vi "ex02.vi"() -> ()   [LabVIEW 2011]
panel:
  in  "stop":bool
  out "Numeric 4":dbl
  out "Numeric 3":i64
  in  "Numeric 2":dbl
  in  "Numeric":i64
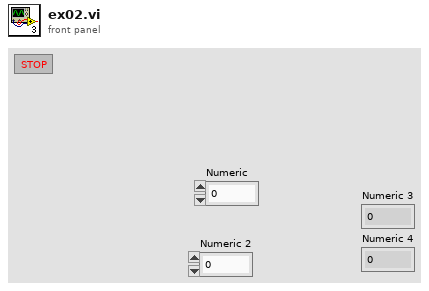
[diagram p1: front panel]
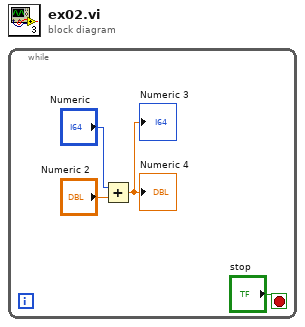
[diagram p0: block diagram]
diagram:
  n1 = while {
    stop <- "stop" stop-if-true
    n2 = Add(x="Numeric", y="Numeric 2") -> (x+y=→"Numeric 3" →"Numeric 4":dbl)
  }
